vi "Actor Core.vi"(8 "error in":errorcluster, 11 "Actor in":refnum<class "Ping Test.lvclass">) -> (0 "error out":errorcluster, 3 "Actor out":refnum<class "Actor.lvclass">)   [LabVIEW 2013, in "Ping Test.lvlib" / "Ping Test.lvclass"]
doc: "This is Actor Core.vi, the main message handling loop for Actors. An actor usually just sits in this loop and processes messages as they arrive. Any error returned by the message Do.vi call will stop the loop, with error code 43 as the cannonical signal to stop with no error sent to caller. Descendants may override that in Handle Error.vi."
uses:
  Ping Test.lvclass
  <vilib>/ActorFramework/Actor/Actor.lvclass
  Ghetto_ping_class/Ghetto_ping.lvclass
  _test class base/_test class base_Actor/_test class base.lvclass
  <vilib>/ActorFramework/Actor/Actor.lvclass/Actor.ctl
  <vilib>/ActorFramework/Message Enqueuer/Message Enqueuer.lvclass/Message Enqueuer.ctl
  _test class base/Messages/Send Status String to UI_Msg/Send Status String to UI_Msg.lvclass/Send Status String to UI_Msg.ctl
  <vilib>/ActorFramework/Message Enqueuer/Init from Existing Queue.vi
  <vilib>/ActorFramework/Message Enqueuer/Enqueue.vi
  <vilib>/ActorFramework/Message Priority Queue/Priority Enqueue.vi
  <vilib>/ActorFramework/Message Enqueuer/Message Enqueuer.lvclass
  _test class base/Messages/Send Status String to UI_Msg/Send Status String to UI_Msg.lvclass
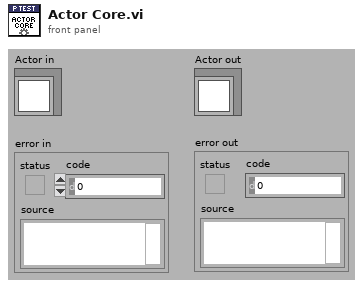
[diagram p1: front panel]
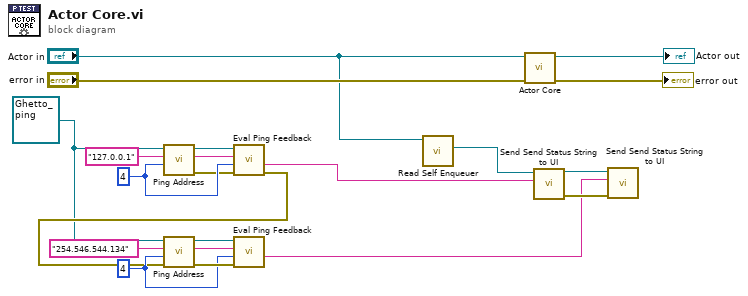
[diagram p0: block diagram]
diagram:
  w12 = 4 ("Number of pings(4)")
  w15 = 4 ("Number of pings(4)")
  w7 = refnum<class "Ghetto_ping.lvclass"> refnum ("object in")
  n1 = call "Ping Address.vi"("Number of pings(4)"=w15, "IP Address(loopback=127.0.0.1)"="127.0.0.1", "object in"=w7) -> ("error out"=w14:errorcluster, "Ping output"=w17:string, "object out"=w18:refnum<class "Ghetto_ping.lvclass">)  [unwired: 5 in, 1 out]
  n2 = call "Eval Ping Feedback.vi"("error in (no error)"=w14, "Pings sent"=w15, "Ping feedback"=w17, "object in"=w18) -> ("error out"=w8:errorcluster, "Report"=w4:string)  [unwired: 4 in, 2 out]
  n3 = call "Ping Address.vi"("error in (no error)"=w8, "Number of pings(4)"=w12, "IP Address(loopback=127.0.0.1)"="254.546.544.134", "object in"=w7) -> ("error out"=w13:errorcluster, "Ping output"=w10:string, "object out"=w9:refnum<class "Ghetto_ping.lvclass">)  [unwired: 4 in, 1 out]
  n4 = call "Eval Ping Feedback.vi"("error in (no error)"=w13, "Pings sent"=w12, "Ping feedback"=w10, "object in"=w9) -> ("Report"=w1:string)  [unwired: 4 in, 3 out]
  n5 = call <vilib>:"Read Self Enqueuer.vi"("Actor"="Actor in") -> ("Self Enqueuer"=w5:refnum<class "Message Enqueuer.lvclass">)  [unwired: 10 in]
  n6 = call-parent "Actor Core.vi"("error in"="error in", "Actor in"="Actor in") -> ("error out"=→"error out":errorcluster, "Actor out"=→"Actor out":refnum<class "Actor.lvclass">)  [unwired: 8 in]
  n7 = call "Send Send Status String to UI.vi"("Status String to Send"=w4, "Message Enqueuer"=w5) -> ("error out"=w2:errorcluster, "Message Enqueuer out"=w3:refnum<class "Message Enqueuer.lvclass">)  [unwired: 8 in]
  n8 = call "Send Send Status String to UI.vi"("error in (no error)"=w2, "Status String to Send"=w1, "Message Enqueuer"=w3) -> ()  [unwired: 7 in, 2 out]
